vi "helper-io-edit.vi"(10 "NewVal":T5(array[cluster]) {"ADDR" format="%04d"; "calibration"."Y" format="%#.1f"}, 11 "OldVal":T5(array[cluster]) {"ADDR" format="%04d"; "calibration"."Y" format="%#.1f"}) -> (0 "error out":errorcluster, 2 "IO changed?":bool, 3 "x != y?":T6(array[cluster]))   [LabVIEW 2024]
uses:
  controls/type.address.ctl
  controls/enum.io.type.ctl
  controls/enum.io.mode.ctl
  controls/typeXyPoint.ctl
  controls/enumVarCtrlIO.ctl
  controls/IONode.ctl
panel:
  out "calibration":cluster{"X":bool, "Y":bool}[](array[cluster])
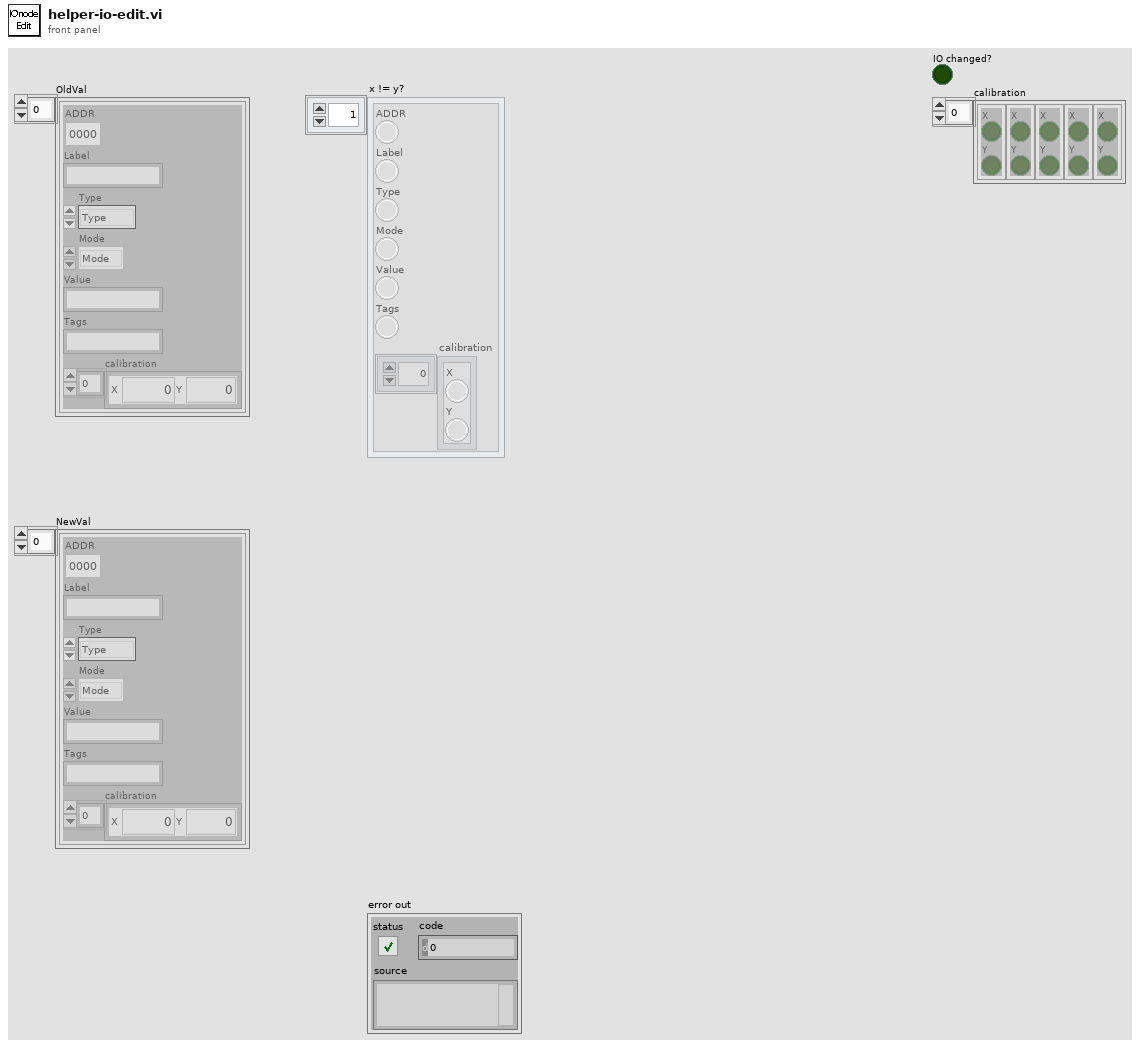
[diagram p1: front panel]
types:
  T1 = typedef "type.address.ctl" = u16
  T2 = typedef "enum.io.type.ctl" = enum16{"Type", "DI", "DO", "AI", "AO", "VL", "BUF"}
  T3 = typedef "enum.io.mode.ctl" = enum16{"Mode", "RIO", "SIM"}
  T4 = typedef "typeXyPoint.ctl" = cluster{"X":dbl, "Y":dbl}
  T5 = cluster{"ADDR":T1, "Label":string, "Type":T2, "Mode":T3, "Value":string, "Tags":string, "calibration":T4[]}[]
  T6 = cluster{"ADDR":bool, "Label":bool, "Type":bool, "Mode":bool, "Value":bool, "Tags":bool, "calibration":cluster{"X":bool, "Y":bool}[]}[]
  T7 = cluster{"ADDR":bool, "Label":bool, "Type":bool, "Mode":bool, "Value":bool, "Tags":bool, "calibration":cluster{"X":bool, "Y":bool}[]}
  T8 = cluster{"ADDR":T1, "Label":string, "Type":T2, "Mode":T3, "Value":string, "Tags":string, "calibration":T4[]}
  T9 = typedef "enumVarCtrlIO.ctl" = enum16{"IO Get By Key", "IO List Configs", "IO Add By Key", "IO Modify Value By Key", "IO Modify Calib By Key", "IO Modify ADDR By Key", "IO Modify Mode By Key", "IO Modify Type By Key", "IO Modify Name By Key", "IO Remove By Key", "IO Remove All"}
  T10 = typedef "IONode.ctl" = cluster{"ADDR":T1, "Label":string, "Type":T2, "Mode":T3, "Value":string, "Tags":string, "calibration":T4[]}
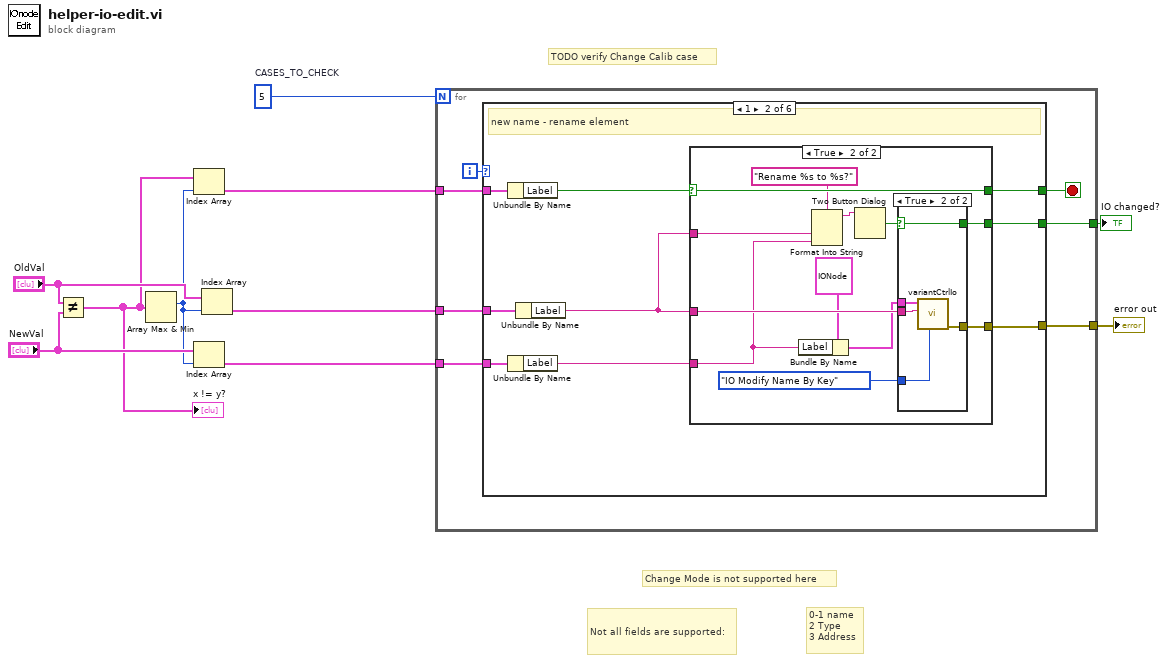
[diagram p0: block diagram]
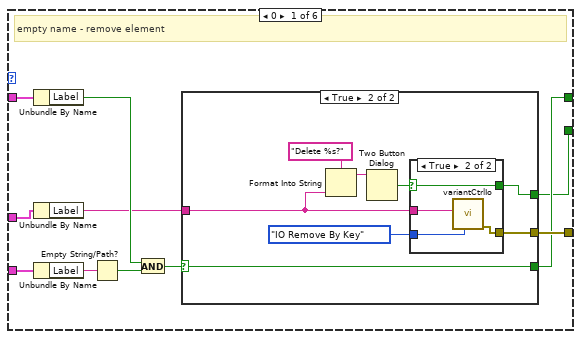
[diagram p2: hidden frame]
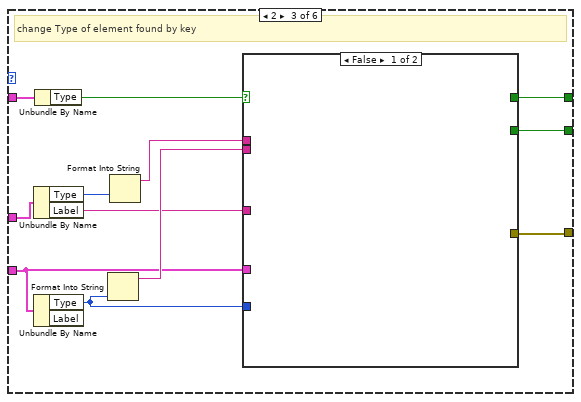
[diagram p7: hidden frame]
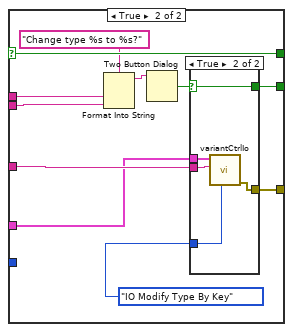
[diagram p8: hidden frame]
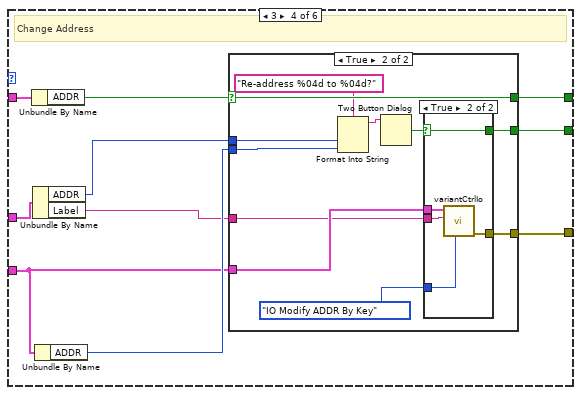
[diagram p10: hidden frame]
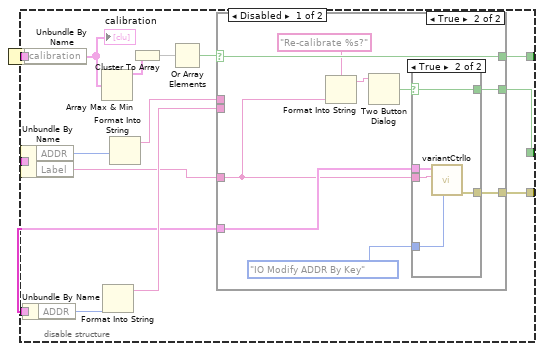
[diagram p14: hidden frame]
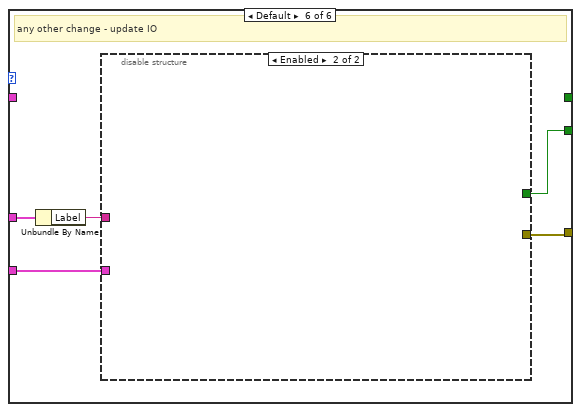
[diagram p17: hidden frame]
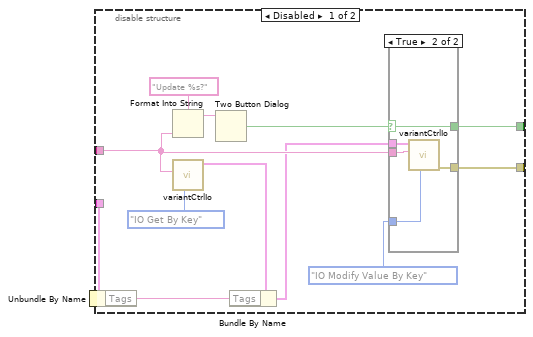
[diagram p18: hidden frame]
diagram:
  w10 = 5  # CASES_TO_CHECK
  # "Not all fields are supported:"
  # "TODO verify Change Calib case"
  # "0-1 name \n2 Type\n3 Address"
  # "Change Mode is not supported here"
  n1 = Not Equal?(x="OldVal", y="NewVal") -> (x != y?=w4:T6)
  "x != y?" <- w4
  n2 = Array Max & Min(array=w4) -> (max index (indices)=w1:i32)  [unwired: 3 out]
  n3 = Index Array(array=w4, index=w1) -> (element=w3:T7)
  n4 = Index Array(array="NewVal", index=w1) -> (element=w7:T8)
  n5 = Index Array(array="OldVal", index=w1) -> (element=w8:T8)
  n6 = for {
    N: w10 -> [_]
    tunnel: w7 -> [w16]
    tunnel: w3 -> [w15]
    tunnel: w8 -> [w11]
    tunnel: [w14] -> w9
    tunnel: [w12] -> w2
    i -> [w17]
    stop <- w13 stop-if-true
    n7 = case shown="1" w17 {
      tunnel: w16 -> [w25 w49 w67 w96 w121 w157]
      tunnel: w15 -> [w24 w48 w78 w104 w126 _]
      tunnel: [w19 w44 w74 w100 w123 _] -> w13
      tunnel: [w21 w47 w77 w103 w125 w160] -> w14
      tunnel: [w18 w43 w73 w99 w122 w156] -> w12
      tunnel: w11 -> [w23 w42 w75 w101 w124 w159]
      frame 0 {
        # "empty name - remove element"
        n8 = Unbundle By Name(w24) -> ("Label"=w28:bool)
        n9 = Unbundle By Name(w23) -> ("Label"=w22:string)
        n10 = Unbundle By Name(w25) -> ("Label"=w26:string)
        n11 = Empty String/Path?(string/path=w26) -> (empty?=w27:bool)
        n12 = And(x=w28, y=w27) -> (x .and. y?=w20:bool)
        n13 = case shown="True" w20 {
          selector: w20 -> [_ w30]
          tunnel: w22 -> [_ w35]
          tunnel: [_ w36] -> w21
          tunnel: [_ w30] -> w19
          tunnel: [_ w29] -> w18
          frame False {
          }
          frame True {
            n14 = Format Into String(format string="Delete %s?", w35) -> (resulting string=w32:string)  [unwired: 2 in, 1 out]
            n15 = Two Button Dialog(message=w32) -> (T button?=w34:bool)  [unwired: 2 in]
            n16 = case shown="True" w34 {
              selector: w34 -> [_ w37]
              tunnel: enumVarCtrlIO."IO Remove By Key" ("menu (Get Param)") -> [_ w40]
              tunnel: w35 -> [_ w39]
              tunnel: [_ w38] -> w36
              tunnel: [_ w37] -> w29
              frame False {
              }
              frame True {
                n17 = call "variantCtrlIo.vi"("menu (Get Param)"=w40, "Key (use IOnode Label if empty )"=w39) -> ("error out"=w38:errorcluster)  [unwired: 5 in, 4 out]
              }
            }
          }
        }
      }
      frame 1 {
        # "new name - rename element"
        n18 = Unbundle By Name(w48) -> ("Label"=w46:bool)
        n19 = Unbundle By Name(w49) -> ("Label"=w45:string)
        n20 = Unbundle By Name(w42) -> ("Label"=w41:string)
        n21 = case shown="True" w46 {
          selector: w46 -> [_ w60]
          tunnel: w45 -> [_ w52]
          tunnel: [_ w61] -> w47
          tunnel: [_ w60] -> w44
          tunnel: w41 -> [_ w55]
          tunnel: [_ w54] -> w43
          tunnel: w41 -> [_ w53]
          frame False {
          }
          frame True {
            n22 = Bundle By Name(cluster=T10 {"ADDR"=0, "Label"="Name", "Type"=enum."DI", "Mode"=enum."RIO", "Value"="Value", "Tags"="Tags", "calibration"=[]} ("input cluster"), "Label"=w52) -> (w50:T10)
            n23 = Format Into String(format string="Rename %s to %s?", w55, w52) -> (resulting string=w57:string)  [unwired: 2 in, 1 out]
            n24 = Two Button Dialog(message=w57) -> (T button?=w59:bool)  [unwired: 2 in]
            n25 = case shown="True" w59 {
              selector: w59 -> [_ w62]
              tunnel: enumVarCtrlIO."IO Modify Name By Key" ("menu (Get Param)") -> [_ w66]
              tunnel: w53 -> [_ w65]
              tunnel: [_ w64] -> w61
              tunnel: w50 -> [_ w63]
              tunnel: [_ w62] -> w54
              frame False {
              }
              frame True {
                n26 = call "variantCtrlIo.vi"("menu (Get Param)"=w66, "Key (use IOnode Label if empty )"=w65, "IOnode in"=w63) -> ("error out"=w64:errorcluster)  [unwired: 4 in, 4 out]
              }
            }
          }
        }
      }
      frame 2 {
        # "change Type of element found by key"
        n27 = Unbundle By Name(w75) -> ("Type"=w72:T2, "Label"=w68:string)
        n28 = Unbundle By Name(w67) -> ("Type"=w69:T2)  [unwired: 1 out]
        n29 = Unbundle By Name(w78) -> ("Type"=w76:bool)
        n30 = Format Into String(w69) -> (resulting string=w70:string)  [unwired: 3 in, 1 out]
        n31 = Format Into String(w72) -> (resulting string=w71:string)  [unwired: 3 in, 1 out]
        n32 = case shown="False" w76 {
          selector: w76 -> [_ w88]
          tunnel: [_ w89] -> w77
          tunnel: [_ w88] -> w74
          tunnel: w71 -> [_ w83]
          tunnel: [_ w82] -> w73
          tunnel: w70 -> [_ w81]
          tunnel: w69 -> [_ _]
          tunnel: w68 -> [_ w80]
          tunnel: w67 -> [_ w79]
          frame False {
          }
          frame True {
            n33 = Format Into String(format string="Change type %s to %s?", w83, w81) -> (resulting string=w85:string)  [unwired: 2 in, 1 out]
            n34 = Two Button Dialog(message=w85) -> (T button?=w87:bool)  [unwired: 2 in]
            n35 = case shown="True" w87 {
              selector: w87 -> [_ w90]
              tunnel: enumVarCtrlIO."IO Modify Type By Key" ("menu (Get Param)") -> [_ w94]
              tunnel: w80 -> [_ w93]
              tunnel: [_ w92] -> w89
              tunnel: w79 -> [_ w91]
              tunnel: [_ w90] -> w82
              frame False {
              }
              frame True {
                n36 = call "variantCtrlIo.vi"("menu (Get Param)"=w94, "Key (use IOnode Label if empty )"=w93, "IOnode in"=w91) -> ("error out"=w92:errorcluster)  [unwired: 4 in, 4 out]
              }
            }
          }
        }
      }
      frame 3 {
        # "Change Address"
        n37 = Unbundle By Name(w104) -> ("ADDR"=w102:bool)
        n38 = Unbundle By Name(w101) -> ("ADDR"=w98:T1, "Label"=w95:string)
        n39 = Unbundle By Name(w96) -> ("ADDR"=w97:T1)
        n40 = case shown="True" w102 {
          selector: w102 -> [_ w114]
          tunnel: w95 -> [_ w108]
          tunnel: [_ w115] -> w103
          tunnel: w96 -> [_ w113]
          tunnel: [_ w114] -> w100
          tunnel: w98 -> [_ w107]
          tunnel: [_ w106] -> w99
          tunnel: w97 -> [_ w105]
          frame False {
          }
          frame True {
            n41 = Format Into String(format string="Re-address %04d to %04d?", w107, w105) -> (resulting string=w110:string)  [unwired: 2 in, 1 out]
            n42 = Two Button Dialog(message=w110) -> (T button?=w112:bool)  [unwired: 2 in]
            n43 = case shown="True" w112 {
              selector: w112 -> [_ w116]
              tunnel: enumVarCtrlIO."IO Modify ADDR By Key" ("menu (Get Param)") -> [_ w120]
              tunnel: w108 -> [_ w119]
              tunnel: [_ w118] -> w115
              tunnel: w113 -> [_ w117]
              tunnel: [_ w116] -> w106
              frame False {
              }
              frame True {
                n44 = call "variantCtrlIo.vi"("menu (Get Param)"=w120, "Key (use IOnode Label if empty )"=w119, "IOnode in"=w117) -> ("error out"=w118:errorcluster)  [unwired: 4 in, 4 out]
              }
            }
          }
        }
      }
      frame 4 {
        # "Change calib"
        n45 = disable-structure shown="Enabled" {
          disable-tunnel: w126 -> [w141 _]
          disable-tunnel: [w140 _] -> w125
          disable-tunnel: w124 -> [w139 _]
          disable-tunnel: [w138 _] -> w123
          disable-tunnel: [w137 _] -> w122
          disable-tunnel: w121 -> [w132 _]
          frame Disabled {
            n46 = Unbundle By Name(w141) -> ("calibration"=w130:cluster{"X":bool, "Y":bool}[])
            "calibration" <- w130
            n47 = Unbundle By Name(w139) -> ("ADDR"=w136:T1, "Label"=w131:string)
            n48 = Unbundle By Name(w132) -> ("ADDR"=w135:T1)
            n49 = Array Max & Min(array=w130) -> (max value=w129:cluster{"X":bool, "Y":bool})  [unwired: 3 out]
            n50 = Format Into String(w135) -> (resulting string=w133:string)  [unwired: 3 in, 1 out]
            n51 = Format Into String(w136) -> (resulting string=w134:string)  [unwired: 3 in, 1 out]
            n52 = Cluster To Array(cluster=w129) -> (array=w128:bool[])
            n53 = Or Array Elements(Boolean array=w128) -> (logical OR=w127:bool)
            n54 = case shown="True" w127 {
              selector: w127 -> [_ w149]
              tunnel: w131 -> [_ w142]
              tunnel: [_ w150] -> w140
              tunnel: w132 -> [_ w148]
              tunnel: [_ w149] -> w138
              tunnel: w134 -> [_ _]
              tunnel: [_ w143] -> w137
              tunnel: w133 -> [_ _]
              frame False {
              }
              frame True {
                n55 = Format Into String(format string="Re-calibrate %s?", w142) -> (resulting string=w145:string)  [unwired: 2 in, 1 out]
                n56 = Two Button Dialog(message=w145) -> (T button?=w147:bool)  [unwired: 2 in]
                n57 = case shown="True" w147 {
                  selector: w147 -> [_ w151]
                  tunnel: enumVarCtrlIO."IO Modify ADDR By Key" ("menu (Get Param)") -> [_ w155]
                  tunnel: w142 -> [_ w154]
                  tunnel: [_ w153] -> w150
                  tunnel: w148 -> [_ w152]
                  tunnel: [_ w151] -> w143
                  frame False {
                  }
                  frame True {
                    n58 = call "variantCtrlIo.vi"("menu (Get Param)"=w155, "Key (use IOnode Label if empty )"=w154, "IOnode in"=w152) -> ("error out"=w153:errorcluster)  [unwired: 4 in, 4 out]
                  }
                }
              }
            }
          }
          frame Enabled {
          }
        }
      }
      frame Default {
        # "any other change - update IO"
        n59 = Unbundle By Name(w159) -> ("Label"=w158:string)
        n60 = disable-structure shown="Enabled" {
          disable-tunnel: [w172 _] -> w160
          disable-tunnel: w158 -> [w166 _]
          disable-tunnel: w157 -> [w163 _]
          disable-tunnel: [w161 _] -> w156
          frame Disabled {
            n61 = Unbundle By Name(w163) -> ("Tags"=w162:string)
            n62 = Format Into String(format string="Update %s?", w166) -> (resulting string=w169:string)  [unwired: 2 in, 1 out]
            n63 = call "variantCtrlIo.vi"("menu (Get Param)"=enumVarCtrlIO."IO Get By Key", "Key (use IOnode Label if empty )"=w166) -> ("IOnode out"=w165:T10)  [unwired: 5 in, 4 out]
            n64 = Two Button Dialog(message=w169) -> (T button?=w171:bool)  [unwired: 2 in]
            n65 = Bundle By Name(cluster=w165, "Tags"=w162) -> (w164:T10)
            n66 = case shown="True" w171 {
              selector: w171 -> [_ w173]
              tunnel: enumVarCtrlIO."IO Modify Value By Key" ("menu (Get Param)") -> [_ w177]
              tunnel: w166 -> [_ w176]
              tunnel: [_ w175] -> w172
              tunnel: w164 -> [_ w174]
              tunnel: [_ w173] -> w161
              frame False {
              }
              frame True {
                n67 = call "variantCtrlIo.vi"("menu (Get Param)"=w177, "Key (use IOnode Label if empty )"=w176, "IOnode in"=w174) -> ("error out"=w175:errorcluster)  [unwired: 4 in, 4 out]
              }
            }
          }
          frame Enabled {
          }
        }
      }
    }
  }
  "error out" <- w9
  "IO changed?" <- w2
